vi "Autonomous Independent.vi"   [LabVIEW 2012]
doc: "This VI is called when autonomous begins, and will automatically be terminated when autonomous ends. You can carry out timed or sensor driven robot movement independently without needing to return to the caller."
uses:
  Robot Global Data.vi
  <vilib>/Rock Robotics/WPI/RobotDrive/WPI_RobotDriveGetSetRefNum.vi
  <vilib>/Rock Robotics/WPI/RobotDrive/WPI_RobotDriveArcadeDrive_Standard(NoSaturation).vi
panel:
  # "Be sure to right-click and choose Data Operations>>Make Current Value default if you want to save the array values with the VI"
types:
  T1 = typedef "WPI_RobotDriveDevRef.ctl" = cluster{"DevStatus":errorcluster, "Motors[]":T2[], "Square Inputs":bool, "Max Output":dbl, "Isochronous":bool}
  T2 = typedef "WPI_MotorControlDeviceRef.ctl" = cluster{"DeviceStatus":errorcluster, "Type":enum16{"PWM", "CAN"}, "PWM":cluster{"Digital Module":T3, "PWM Channel":T4, "DeadBand":T5}, "CAN":cluster{"Device Number":u8, "Control Mode":T6, "Semaphore":T7, "Max Vout":dbl}, "Invert":bool, "TransformRef":T8, "InvTransformRef":T8}
  T3 = typedef "FPGA_TypedefDigitalModule.ctl" = enum16{"Digital Module 1", "Digital Module 2"}
  T4 = typedef "FPGA_DIOPWMChannel.ctl" = enum8{"PWM 1", "PWM 2", "PWM 3", "PWM 4", "PWM 5", "PWM 6", "PWM 7", "PWM 8", "PWM 9", "PWM 10", "Invalid"}
  T5 = typedef "WPI_PWMDeadband.ctl" = cluster{"Name":string, "maxPositivePwm":i32, "minPositivePwm":i32, "centerPwm":i32, "maxNegativePwm":i32, "minNegativePwm":i32, "angularRange":u16}
  T6 = typedef "WPI_CANJaguar_ControlMode.ctl" = enum8{"Percent VBus", "Current", "Speed", "Position", "Voltage"}
  T7 = typedef "Semaphore RefNum" = refnum<k1>
  T8 = typedef "WPI_PWMTransform_ConPane.ctl" = refnum<vi>
  T9 = cluster{"Center Position":cluster{"X":dbl, "Y":dbl}, "Distance (ft)":dbl, "Center":bool}[]
  T10 = cluster{"Center Position":cluster{"X":dbl, "Y":dbl}, "Distance (ft)":dbl, "Center":bool}
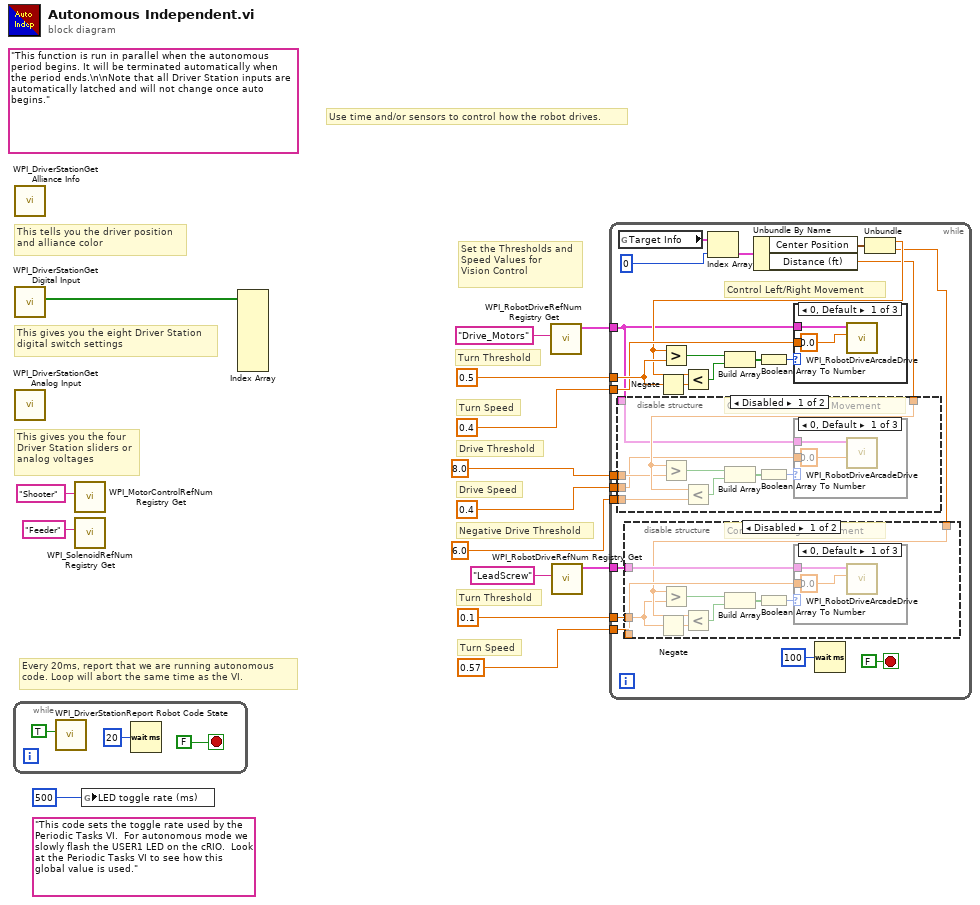
[diagram p0: block diagram]
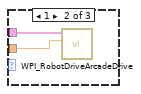
[diagram p2: hidden frame]
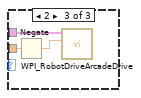
[diagram p3: hidden frame]
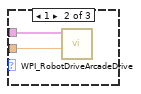
[diagram p5: hidden frame]
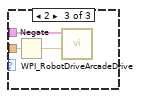
[diagram p6: hidden frame]
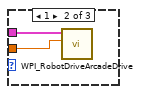
[diagram p8: hidden frame]
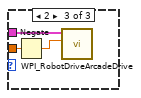
[diagram p9: hidden frame]
diagram:
  (unwired) "This code sets the toggle rate used by the Periodic Tasks VI.  For autonomous mode we slowly flash the USER1 LED on the cRIO.  Look at the Periodic Tasks VI to see how this global value is used."
  (unwired) "This function is run in parallel when the autonomous period begins. It will be terminated automatically when the period ends.\n\nNote that all Driver Station inputs are automatically latched and will not change once auto begins."
  # "Turn Threshold"
  # "Turn Speed"
  # "Set the Thresholds and\nSpeed Values for\nVision Control"
  # "Negative Drive Threshold"
  # "Drive Threshold"
  # "Drive Speed"
  # "Turn Threshold"
  # "Turn Speed"
  # "Every 20ms, report that we are running autonomous\ncode. Loop will abort the same time as the VI."
  # "Use time and/or sensors to control how the robot drives."
  # "This tells you the driver position\nand alliance color"
  # "This gives you the eight Driver Station\ndigital switch settings"
  # "This gives you the four\nDriver Station sliders or\nanalog voltages"
  n1 = while {
    stop <- FALSE stop-if-true
    n2 = call <vilib>:"WPI_DriverStationReport Robot Code State.vi"("Autonomous"=TRUE) -> ()  [unwired: 10 in, 1 out]
    n3 = Wait (ms)(milliseconds to wait=u32 20) -> ()  [unwired: 1 out]
  }
  n4 = call <vilib>:"WPI_DriverStationGet Alliance Info.vi"() -> ()  [unwired: 12 out]
  n5 = call <vilib>:"WPI_DriverStationGet Digital Input.vi"() -> ("Driver Station Digital Input (1-8)"=w15:bool[])  [unwired: 11 out]
  n6 = call <vilib>:"WPI_DriverStationGet Analog Input.vi"() -> ()  [unwired: 12 out]
  n7 = call <vilib>:"WPI_MotorControlRefNum Registry Get.vi"("refnum name"="Shooter") -> ()  [unwired: 9 in, 2 out]
  n8 = call <vilib>:"WPI_SolenoidRefNum Registry Get.vi"("refnum name"="Feeder") -> ()  [unwired: 9 in, 2 out]
  n9 = global write "Robot Global Data.vi" "LED toggle rate (ms)"(u32 500 ("LED ms toggle rate")) -> ()
  n10 = Index Array(array=w15) -> ()  [unwired: 8 in, 8 out]
  n11 = call <vilib>:"WPI_RobotDriveRefNum Registry Get.vi"("refnum name"="Drive_Motors") -> ("RobotDriveDevRef"=w6:T1)  [unwired: 9 in, 1 out]
  n12 = call <vilib>:"WPI_RobotDriveRefNum Registry Get.vi"("refnum name"="LeadScrew") -> ("RobotDriveDevRef"=w3:T1)  [unwired: 9 in, 1 out]
  n13 = while {
    tunnel: w6 -> [w24]
    tunnel: 0.4 -> [w31]
    tunnel: 0.5 ("y") -> [w36]
    tunnel: 8.0 ("y") -> [w26]
    tunnel: 0.4 -> [w25]
    tunnel: 6.0 -> [w23]
    tunnel: w3 -> [w22]
    tunnel: 0.1 ("y") -> [w19]
    tunnel: 0.57 -> [w21]
    stop <- FALSE stop-if-true
    # "Control Left/Right Movement"
    n14 = global read "Robot Global Data.vi" "Target Info"() -> (w41:T9)
    n15 = Negate(x=w36) -> (-x=w37:dbl)
    n16 = Index Array(array=w41, index=0) -> (element=w39:T10)
    n17 = Unbundle By Name(w39) -> ("Center Position"=w29:cluster{"X":dbl, "Y":dbl}, "Distance (ft)"=w27:dbl)
    n18 = disable-structure shown="Disabled" {
      disable-tunnel: w27 -> [w63 _]
      disable-tunnel: w26 -> [w62 _]
      disable-tunnel: w25 -> [w60 _]
      disable-tunnel: w24 -> [w59 _]
      disable-tunnel: w23 -> [w58 _]
      frame Disabled {
        # "Control Forward/Back Movement"
        n19 = Greater?(x=w63, y=w62) -> (0:w66:bool)
        n20 = Less?(x=w63, y=w58) -> (x < y?=w65:bool)
        n21 = Build Array(w66, w65) -> (w64:bool[])
        n22 = Boolean Array To Number(Boolean array=w64) -> (number=w61:u32)
        n23 = case shown="0, Default" w61 {
          tunnel: w59 -> [w68 w70 w72]
          tunnel: w60 -> [_ w69 w73]
          frame 0, Default {
            n24 = call-poly <vilib>:"WPI_RobotDriveArcadeDrive.vi"("Y axis value"=0.0 ("X axis value"), "RobotDriveDevRef"=w68) -> ()  [unwired: 7 in, 3 out]
          }
          frame 1 {
            n25 = call-poly <vilib>:"WPI_RobotDriveArcadeDrive.vi"("Y axis value"=w69, "RobotDriveDevRef"=w70) -> ()  [unwired: 7 in, 3 out]
          }
          frame 2 {
            n26 = Negate(x=w73) -> (-x=w71:dbl)
            n27 = call-poly <vilib>:"WPI_RobotDriveArcadeDrive.vi"("Y axis value"=w71, "RobotDriveDevRef"=w72) -> ()  [unwired: 7 in, 3 out]
          }
        }
      }
      frame Enabled {
      }
    }
    n28 = Wait (ms)(milliseconds to wait=u32 100) -> ()  [unwired: 1 out]
    n29 = Unbundle(w29) -> ("X"=w28:dbl, "Y"=w20:dbl)
    n30 = disable-structure shown="Disabled" {
      disable-tunnel: w22 -> [w45 _]
      disable-tunnel: w21 -> [w44 _]
      disable-tunnel: w20 -> [w43 _]
      disable-tunnel: w19 -> [w42 _]
      frame Disabled {
        # "Control Left/Right Movement"
        n31 = Negate(x=w42) -> (-x=w50:dbl)
        n32 = Greater?(x=w43, y=w42) -> (0:w49:bool)
        n33 = Less?(x=w43, y=w50) -> (x < y?=w48:bool)
        n34 = Build Array(w49, w48) -> (w47:bool[])
        n35 = Boolean Array To Number(Boolean array=w47) -> (number=w46:u32)
        n36 = case shown="0, Default" w46 {
          tunnel: w45 -> [w52 w54 w56]
          tunnel: w44 -> [_ w53 w57]
          frame 0, Default {
            n37 = call-poly <vilib>:"WPI_RobotDriveArcadeDrive.vi"("X axis value"=0.0, "RobotDriveDevRef"=w52) -> ()  [unwired: 7 in, 3 out]
          }
          frame 1 {
            n38 = call-poly <vilib>:"WPI_RobotDriveArcadeDrive.vi"("X axis value"=w53, "RobotDriveDevRef"=w54) -> ()  [unwired: 7 in, 3 out]
          }
          frame 2 {
            n39 = Negate(x=w57) -> (-x=w55:dbl)
            n40 = call-poly <vilib>:"WPI_RobotDriveArcadeDrive.vi"("X axis value"=w55, "RobotDriveDevRef"=w56) -> ()  [unwired: 7 in, 3 out]
          }
        }
      }
      frame Enabled {
      }
    }
    n41 = Greater?(x=w28, y=w36) -> (0:w35:bool)
    n42 = Less?(x=w28, y=w37) -> (x < y?=w34:bool)
    n43 = Build Array(w35, w34) -> (w33:bool[])
    n44 = Boolean Array To Number(Boolean array=w33) -> (number=w32:u32)
    n45 = case shown="0, Default" w32 {
      tunnel: w24 -> [w75 w77 w79]
      tunnel: w31 -> [_ w76 w80]
      frame 0, Default {
        n46 = call-poly <vilib>:"WPI_RobotDriveArcadeDrive.vi"("X axis value"=0.0, "RobotDriveDevRef"=w75) -> ()  [unwired: 7 in, 3 out]
      }
      frame 1 {
        n47 = call-poly <vilib>:"WPI_RobotDriveArcadeDrive.vi"("X axis value"=w76, "RobotDriveDevRef"=w77) -> ()  [unwired: 7 in, 3 out]
      }
      frame 2 {
        n48 = Negate(x=w80) -> (-x=w78:dbl)
        n49 = call-poly <vilib>:"WPI_RobotDriveArcadeDrive.vi"("X axis value"=w78, "RobotDriveDevRef"=w79) -> ()  [unwired: 7 in, 3 out]
      }
    }
  }
